vi "_macro_Choreo_GetTrajectory.vi"() -> ()   [LabVIEW 2019, in "ChoreoLib.lvlib"]
uses:
  ChoreoLib.lvlib
  TypeDef/ChoreoTrajectory.ctl
  TypeDef/ChoreoTrajectoryState.ctl
panel:
  out "ChoreoTrajectory":T1
  out "error out":errorcluster
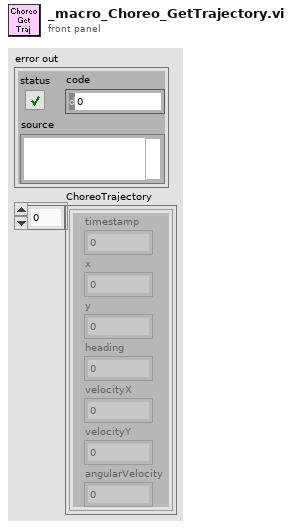
[diagram p1: front panel]
types:
  T1 = typedef "ChoreoLib.lvlib/ChoreoTrajectory.ctl" = T2[]
  T2 = typedef "ChoreoLib.lvlib/ChoreoTrajectoryState.ctl" = cluster{"timestamp":dbl, "x":dbl, "y":dbl, "heading":dbl, "velocityX":dbl, "velocityY":dbl, "angularVelocity":dbl}
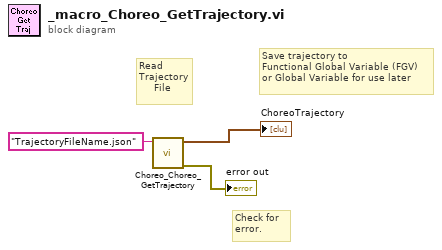
[diagram p0: block diagram]
diagram:
  # "Save trajectory to\nFunctional Global Variable (FGV)\nor Global Variable for use later"
  # "Check for \nerror."
  # "Read\nTrajectory\n     File"
  n1 = call "Choreo_Choreo_GetTrajectory.vi"("FileName"="TrajectoryFileName.json") -> ("error out"=→"error out":errorcluster, "ChoreoTrajectory"=→"ChoreoTrajectory":T1)  [unwired: 8 in, 1 out]
